vi "processFile.vi"(7 "error in":errorcluster, 10 "selected path":path) -> (0 "error out":errorcluster, 1 "numberSignals":u32, 2 "resolution":u32, 3 "readyData":u32[](array[numeric])=[10, 10, 10, 10, 10, 10, 10, 10, 10, 10, 10, 10, 10, 10, 10, 10, 4294967295, 0, 4294967295, 0, 4294967295, 0, 4294967295, 0, 4294967295, 0, 4294967295, 0, 4294967295, 0, 4294967295, 0, 65535] format="%x")   [LabVIEW 2014]
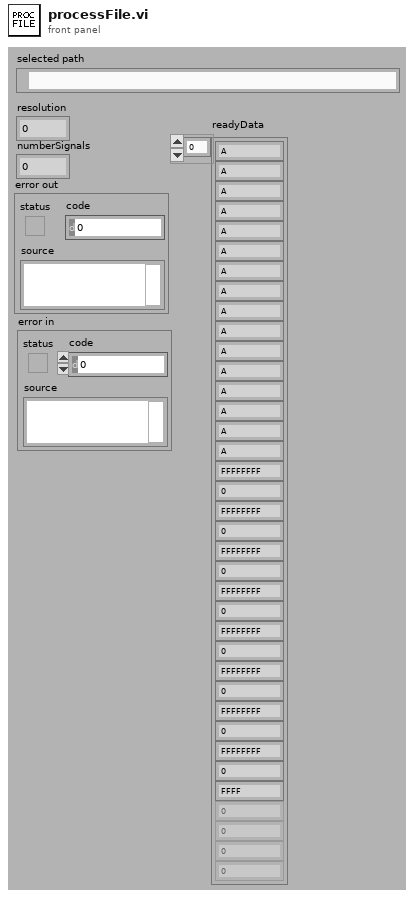
[diagram p1: front panel]
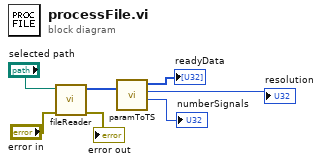
[diagram p0: block diagram]
diagram:
  n1 = call "fileReader.vi"("error in"="error in", "filepath"="selected path") -> ("error out"=→"error out":errorcluster, "dataout"=w5:u32[])  [unwired: 8 out]
  n2 = call "paramToTS.vi"("dataout"=w5) -> ("numberSignals"=→"numberSignals":u32, "resolution"=→"resolution":u32, "readyData"=→"readyData":u32[])  [unwired: 8 out]
